vi "LoadOrCreateAParaIniCfg.vi"(8 "error in":errorcluster, 10 "Tree Refnum":refnum<vi>, 11 "Tbl Refnum in":refnum<vi>) -> (0 "error out":errorcluster, 1 "cfg file refnum out":refnum<file>, 2 "Tree Refnum out":refnum<vi>, 3 "Tbl Refnum out":refnum<vi>)   [LabVIEW 2010]
panel:
  out "All Tags":string[](array[string])
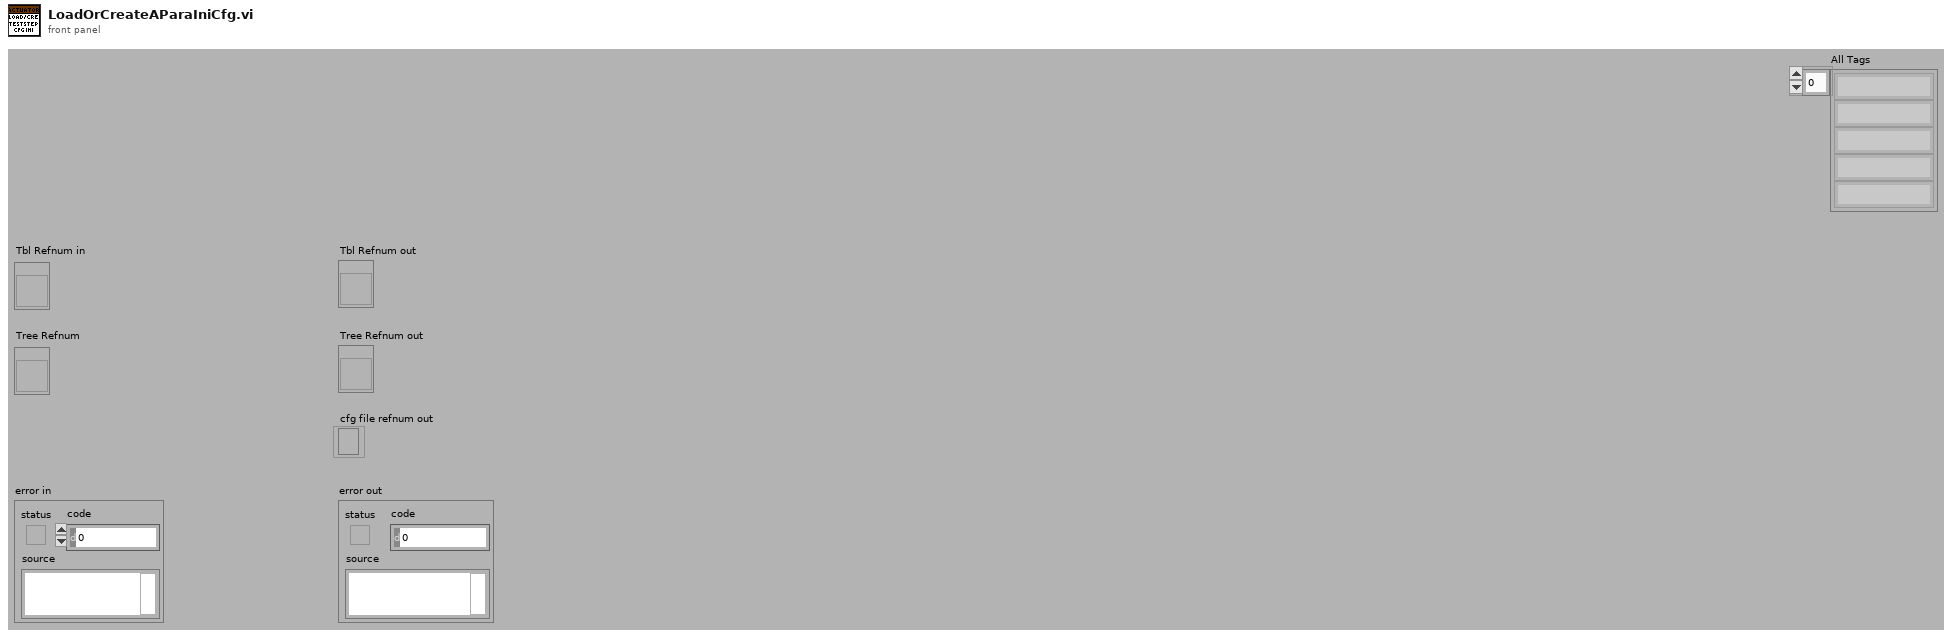
[diagram p1: front panel]
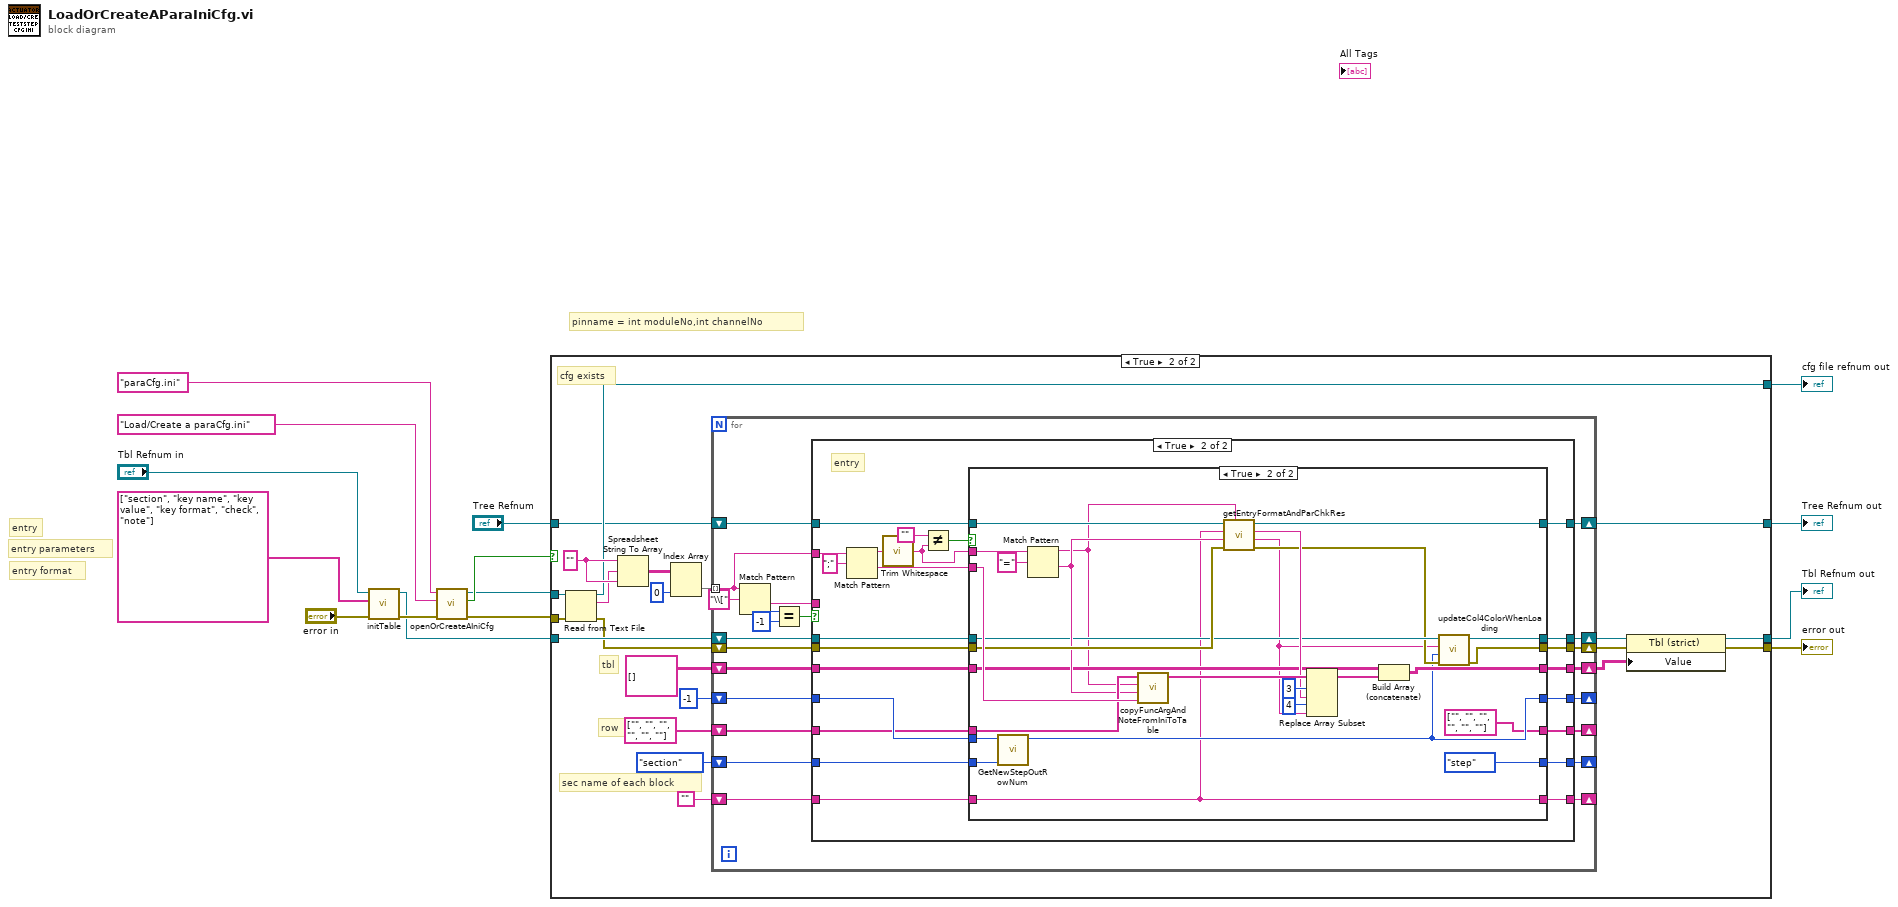
[diagram p0: block diagram]
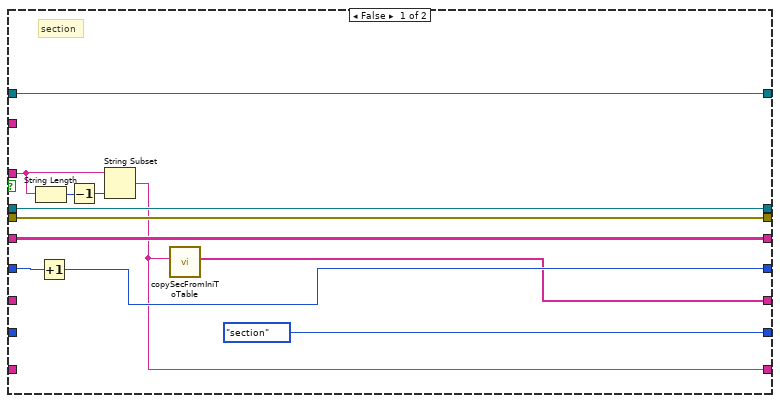
[diagram p3: hidden frame]
diagram:
  # "entry format"
  # "entry parameters"
  # "entry"
  # "pinname = int moduleNo,int channelNo"
  n1 = call "initTable.vi"("error in"="error in", "Column Header Strings[]"=string[] ["section", "key name", "key value", "key format", "check", "note"] ("Row Header Strings[]"), "Tbl Refnum in"="Tbl Refnum in") -> ("error out"=w8:errorcluster, "Tbl Refnum out"=w4:refnum<vi>)  [unwired: 7 in]
  n2 = call "openOrCreateAIniCfg.vi"("error in"=w8, "prompt"="Load/Create a paraCfg.ini", "default name"="paraCfg.ini" ("prompt")) -> ("error out"=w5:errorcluster, "exists"=w7:bool, "ini refnum out"=w6:refnum<file>)  [unwired: 6 in]
  n3 = case shown="True" w7 {
    tunnel: w6 -> [w19 w37]
    tunnel: w5 -> [w18 w36]
    tunnel: w4 -> [w17 w34]
    tunnel: [w19 w31] -> w15
    tunnel: [w18 w20] -> w14
    tunnel: [w17 w21] -> w13
    tunnel: "Tree Refnum" -> [w16 w29]
    tunnel: [w16 w28] -> w11
    frame False {
      # "create a new cfg"
    }
    frame True {
      w39 = ""
      # "sec name of each block"
      # "row"
      # "tbl"
      # "cfg exists"
      n4 = Read from Text File(file (use dialog)=w37, error in=w36) -> (refnum out=w31:refnum<file>, text=w38:string, error out=w30:errorcluster)  [unwired: 2 in, 1 out]
      n5 = Spreadsheet String To Array(format string=w39, spreadsheet string=w38, array type (2D Dbl)=w39) -> (array=w40:string[][])  [unwired: 1 in]
      n6 = Index Array(array=w40, index (col)=0 ("disabled index (col)")) -> (element=w35:string[])  [unwired: 1 in]
      n7 = for {
        tunnel: w35 -> [w57] mode=indexing
        shift-right: [w55] -> _
        shift-left: -1 -> [w59]
        shift-right: [w54] -> _
        shift-left: enum16{"section", "step"}."section" -> [w53]
        shift-right: [w52] -> w23
        shift-left: w30 -> [w51]
        shift-right: [w50] -> w24
        shift-left: w34 -> [w56]
        shift-right: [w48] -> w28
        shift-left: w29 -> [w49]
        shift-right: [w45] -> w22
        shift-left: string[][] [] -> [w46]
        shift-right: [w47] -> _
        shift-left: string[] ["", "", "", "", "", ""] -> [w42]
        shift-right: [w43] -> _
        shift-left: "" -> [w44]
        n8 = Match Pattern(string=w57, regular expression="\\[") -> (after substring=w58:string, offset past match=w62:i32)  [unwired: 1 in, 2 out]
        n9 = Equal?(x=w62, y=-1) -> (x = y?=w60:bool)
        n10 = case shown="True" w60 {
          tunnel: w59 -> [w72 w97]
          tunnel: [w71 w96] -> w55
          tunnel: w58 -> [w75 _]
          tunnel: w57 -> [_ w90]
          tunnel: w56 -> [w67 w98]
          tunnel: [enum16{"section", "step"}."section" w95] -> w54
          tunnel: w53 -> [_ w94]
          tunnel: w51 -> [w68 w93]
          tunnel: [w68 w92] -> w52
          tunnel: [w67 w91] -> w50
          tunnel: w49 -> [w69 w86]
          tunnel: [w69 w88] -> w48
          tunnel: [w66 w77] -> w47
          tunnel: w46 -> [w65 w79]
          tunnel: [w65 w78] -> w45
          tunnel: w44 -> [_ w80]
          tunnel: [w64 w76] -> w43
          tunnel: w42 -> [_ w81]
          frame False {
            # "section"
            n11 = String Length(string=w75) -> (length=w74:i32)
            n12 = Increment(x=w72) -> (x+1=w71:i32)
            n13 = Decrement(x=w74) -> (x-1=w73:i32)
            n14 = String Subset(string=w75, length (rest)=w73) -> (substring=w64:string)  [unwired: 1 in]
            n15 = call "copySecFromIniToTable.vi"("valInCol0"=w64) -> ("arrWithSec"=w66:string[])  [unwired: 10 in]
          }
          frame True {
            # "entry"
            n16 = Match Pattern(string=w90, regular expression=";") -> (before substring=w85:string, after substring=w87:string)  [unwired: 1 in, 2 out]
            n17 = call <vilib>:"Trim Whitespace.vi"("string"=w85) -> ("trimmed string"=w82:string)  [unwired: 1 in]
            n18 = Not Equal?(x="", y=w82) -> (x != y?=w83:bool)
            n19 = case shown="True" w83 {
              tunnel: w98 -> [w103 w116]
              tunnel: w97 -> [w106 w133]
              tunnel: [w106 w111] -> w96
              tunnel: [w105 enum16{"section", "step"}."step"] -> w95
              tunnel: w94 -> [w105 w132]
              tunnel: w93 -> [w104 w126]
              tunnel: [w104 w114] -> w92
              tunnel: [w103 w113] -> w91
              tunnel: [w102 w124] -> w88
              tunnel: w87 -> [_ w129]
              tunnel: w86 -> [w102 w127]
              tunnel: w82 -> [_ w130]
              tunnel: w81 -> [w101 w128]
              tunnel: w80 -> [w99 w108]
              tunnel: w79 -> [w100 w118]
              tunnel: [w100 w117] -> w78
              tunnel: [w101 string[] ["", "", "", "", "", ""]] -> w77
              tunnel: [w99 w108] -> w76
              frame False {
                # "blank"
              }
              frame True {
                n20 = call "GetNewStepOutRowNum.vi"("lastStat"=w132, "lastRowNum"=w133) -> ("outRowNum"=w111:i32)  [unwired: 9 in]
                n21 = Match Pattern(string=w130, regular expression="=") -> (before substring=w107:string, after substring=w125:string)  [unwired: 1 in, 2 out]
                n22 = call "copyFuncArgAndNoteFromIniToTable.vi"("valInCol5"=w129, "valInCol2"=w125, "valInCol1"=w107, "arrayAtTheSameRow"=w128) -> ("arrWithFunc&Arg&Note"=w123:string[])  [unwired: 7 in]
                n23 = call "getEntryFormatAndParChkRes.vi"("entryName"=w107, "error in"=w126, "arg"=w125, "sec"=w108, "Tree Refnum in"=w127) -> ("error out"=w115:errorcluster, "Check result"=w112:string, "entryFormat"=w120:string, "Tree Refnum out"=w124:refnum<vi>)  [unwired: 3 in]
                n24 = Replace Array Subset(array=w123, new element #1=w120, index #1=3 ("index"), new element #2=w112, index #2=4 ("index")) -> (w119:string[])
                n25 = Build Array (concatenate)(w118, w119) -> (w117:string[][])
                n26 = call "updateCol4ColorWhenLoading.vi"("error in"=w115, "rowNum"=w111, "judgeRes"=w112, "Tbl Refnum in"=w116) -> ("error out"=w114:errorcluster, "Tbl Refnum Out"=w113:refnum<vi>)  [unwired: 6 in]
              }
            }
          }
        }
      }
      n27 = property class="Tbl (strict)"(reference=w24, error in=w23, "Value"=w22) -> (reference out=w21:refnum<vi>, error out=w20:errorcluster)
    }
  }
  "error out" <- w14
  "cfg file refnum out" <- w15
  "Tbl Refnum out" <- w13
  "Tree Refnum out" <- w11
